vi "SetReference.vi"(8 "error in (no error)":errorcluster, 10 "SceneObject":refnum<vi>) -> (0 "error out":errorcluster, 3 "3D Object out":refnum<class "3D Object.lvclass">)   [LabVIEW 2015, in "3D Object.lvclass"]
uses:
  3D Object.lvclass
  3D Object.lvclass/3D Object.ctl
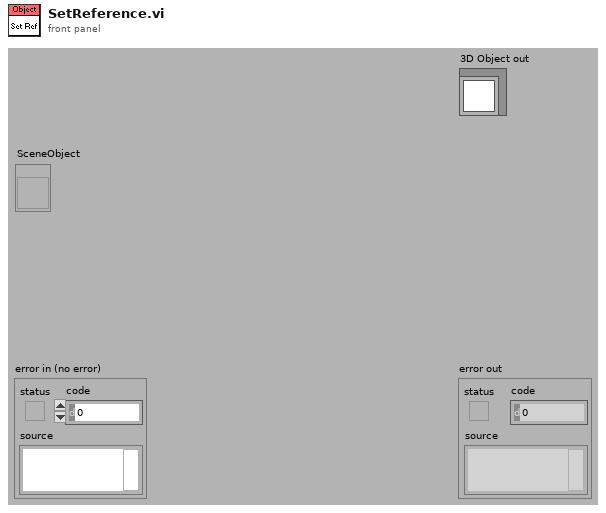
[diagram p1: front panel]
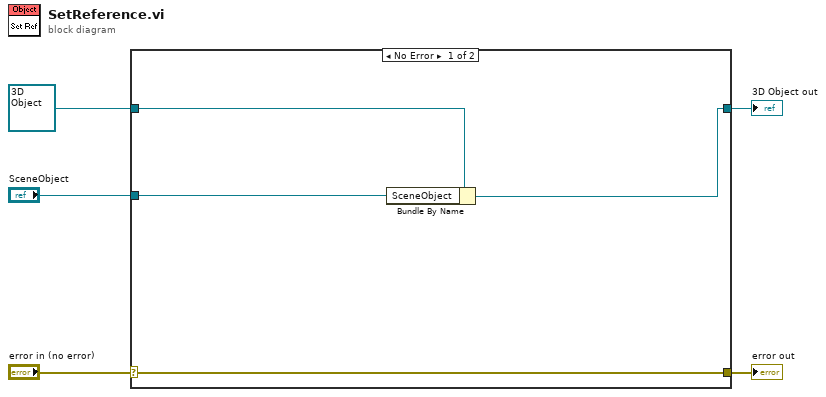
[diagram p0: block diagram]
diagram:
  n1 = case shown="No Error" "error in (no error)" {
    selector: "error in (no error)" -> [w9 w11]
    tunnel: [w9 w11] -> w4
    tunnel: [w7 w10] -> w2
    tunnel: refnum<class "3D Object.lvclass"> refnum ("3D Object in") -> [w8 w10]
    tunnel: "SceneObject" -> [w6 _]
    frame No Error {
      n2 = Bundle By Name(cluster=w8, "SceneObject"=w6) -> (w7:refnum<class "3D Object.lvclass">)
    }
    frame Error {
    }
  }
  "error out" <- w4
  "3D Object out" <- w2
